vi "Waveform Averaging Example.vi"() -> ()   [LabVIEW 2012]
uses:
  <vilib>/measure/NI_MABase.lvlib
panel:
  out "Averaged Waveform 2":waveform(dbl)(graph)
  out "Averaged Waveform":waveform(dbl)(graph)
  in  "Samples to Average":i32=10 min=1
  in  "Stop":bool
  out "Noisy Waveform":waveform(dbl)(graph)
  in  "Amplitude":dbl=10.0 format="%0.2p"
  in  "Frequency":dbl=3.0 format="%0.2p"
  in  "Signal Type":T1(ring)
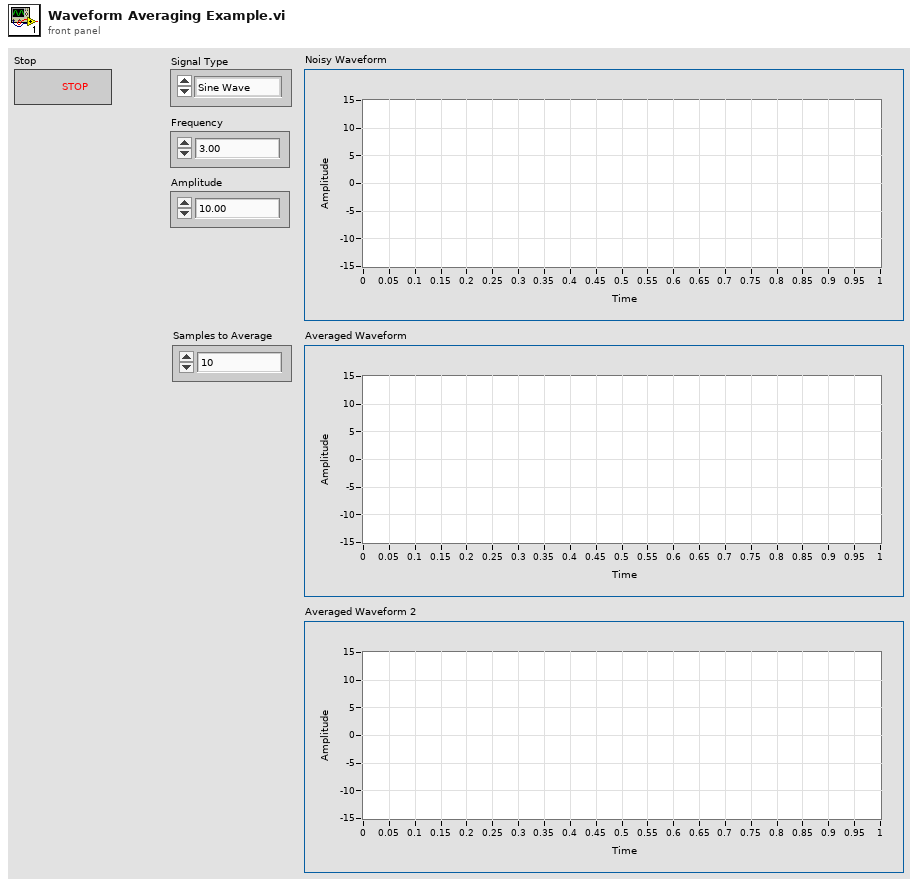
[diagram p1: front panel]
types:
  T1 = enum16{"Sine Wave", "Triangle Wave", "Square Wave", "Sawtooth Wave"}
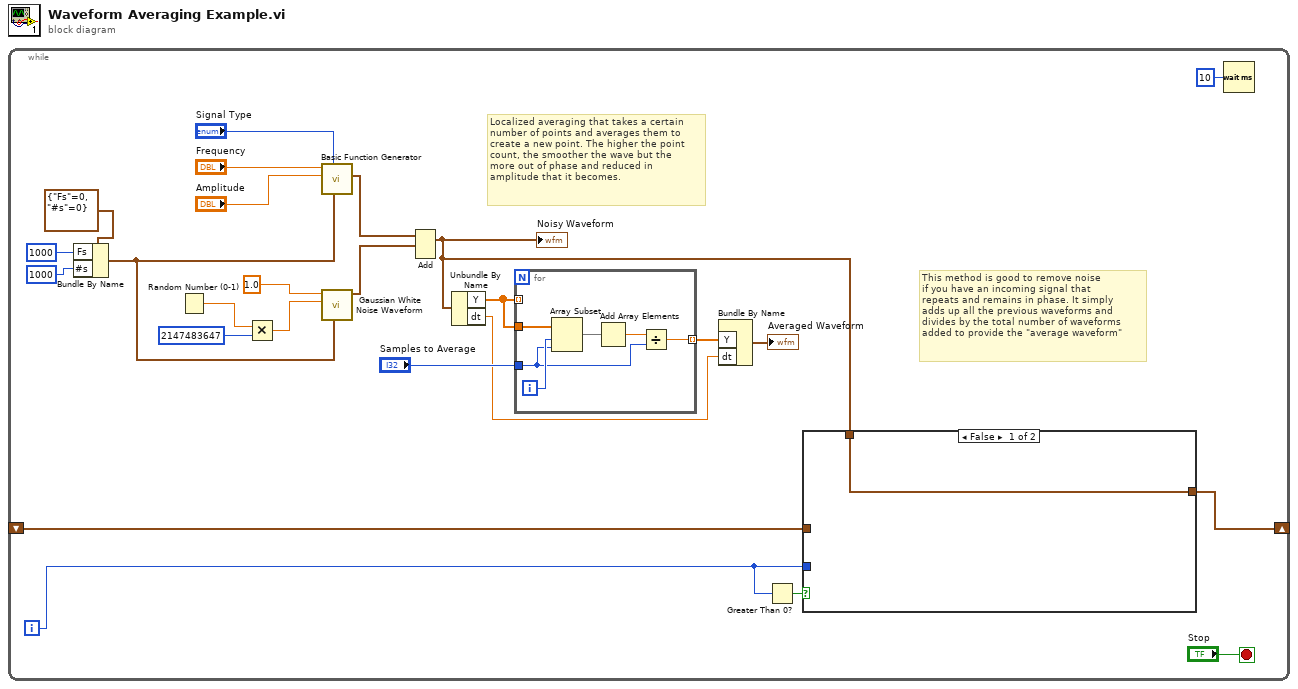
[diagram p0: block diagram]
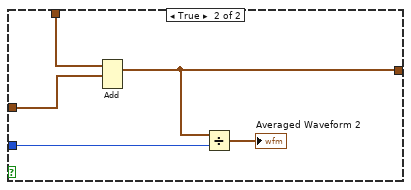
[diagram p2: hidden frame]
diagram:
  n1 = while {
    shift-right: [w4] -> _
    shift-left: _ -> [w5]
    i -> [w1]
    stop <- "Stop" stop-if-true
    # "Localized averaging that takes a certain\nnumber of points and averages them to\ncreate a new point. The higher the point \ncount, the smoother the wave but the \nmore out of phase and reduced in \namplitude that it becomes."
    # "This method is good to remove noise\nif you have an incoming signal that \nrepeats and remains in phase. It simply \nadds up all the previous waveforms and \ndivides by the total number of waveforms \nadded to provide the \"average waveform\""
    n2 = Bundle By Name(cluster=cluster{"Fs":i32, "#s":i32} {"Fs"=0, "#s"=0}, "Fs"=1000, "#s"=1000) -> (w17:cluster{"Fs":i32, "#s":i32})
    n3 = Random Number (0-1)() -> (number: 0 to 1=w22:dbl)
    n4 = Multiply(x=w22, y=2147483647) -> (x*y=w20:dbl)
    n5 = call <vilib>:"Basic Function Generator.vi"("sampling info"=w17, "signal type"="Signal Type", "amplitude"="Amplitude", "frequency"="Frequency") -> ("signal out"=w14:waveform(dbl))  [unwired: 5 in, 2 out]
    n6 = call <vilib>:"Gaussian White Noise Waveform.vi"("sampling info"=w17, "seed"=w20, "standard deviation"=1.0) -> ("signal out"=w13:waveform(dbl))  [unwired: 7 in, 1 out]
    n7 = Add(1:w13, 2:w14) -> (0:w3:waveform(dbl))  [unwired: 1 in, 1 out]
    "Noisy Waveform" <- w3
    n8 = Unbundle By Name(w3) -> ("Y"=w10:dbl[], "dt"=w6:dbl)
    n9 = for {
      tunnel: w10 -> [_] mode=indexing
      tunnel: w10 -> [w37]
      tunnel: "Samples to Average" -> [w33]
      tunnel: [w32] -> w7 mode=indexing
      i -> [w36]
      n10 = Array Subset(array=w37, index=w36, length=w33) -> (w35:dbl[])
      n11 = Add Array Elements(numeric array=w35) -> (sum=w34:dbl)
      n12 = Divide(x=w34, y=w33) -> (x/y=w32:dbl)
    }
    n13 = Bundle By Name("Y"=w7, "dt"=w6) -> (→"Averaged Waveform":waveform(dbl))  [unwired: 1 in]
    n14 = Greater Than 0?(x=w1) -> (x > 0?=w2:bool)
    n15 = case shown="False" w2 {
      tunnel: w5 -> [_ w31]
      tunnel: [w26 w30] -> w4
      tunnel: w1 -> [_ w29]
      tunnel: w3 -> [w26 w28]
      frame False {
      }
      frame True {
        n16 = Add(1:w31, 2:w28) -> (0:w30:waveform(dbl))  [unwired: 1 in, 1 out]
        n17 = Divide(x=w30, y=w29) -> (x/y=→"Averaged Waveform 2":waveform(dbl))
      }
    }
    n18 = Wait (ms)(milliseconds to wait=u32 10) -> ()  [unwired: 1 out]
  }
